vi "Replace Embedded SVG.vi"(7 "image":T1, 8 "error in":errorcluster, 9 "xlink:href":string, 10 "XML In":string, 11 "SVGImage in":refnum<class "SVGImage.lvclass">) -> (0 "error out":errorcluster, 2 "Edited XML Out":string, 3 "SVGImage out":refnum<class "SVGImage.lvclass">)   [LabVIEW 2019, in "SVGImage.lvclass"]
uses:
  SVGImage.lvclass
  ParseXML/Image.ctl
  SVGImage.lvclass/SVGImage.ctl
  EditSVG/EditSVG.lvclass
  ParseXML/ParseSVG.lvclass
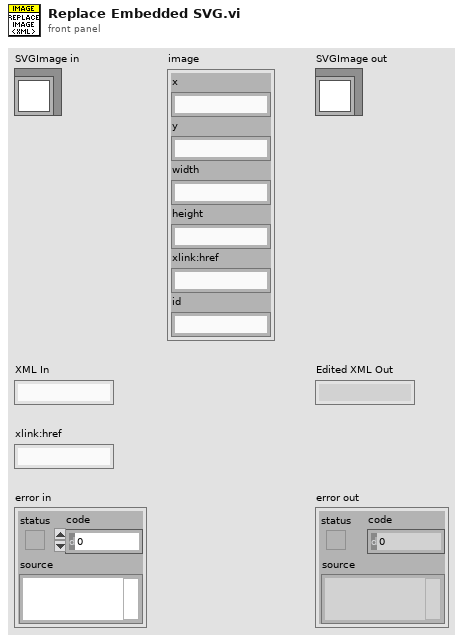
[diagram p1: front panel]
types:
  T1 = typedef "ParseSVG.lvclass/Image.ctl" = cluster{"x":string, "y":string, "width":string, "height":string, "xlink:href":string, "id":string}
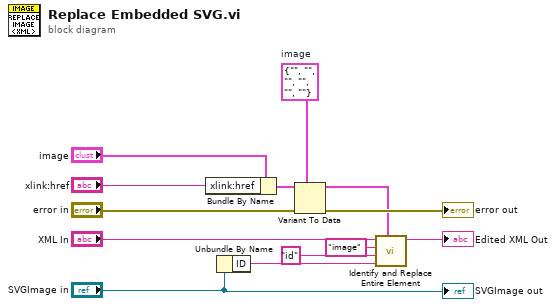
[diagram p0: block diagram]
diagram:
  w13 = T1 {"x"="", "y"="", "width"="", "height"="", "xlink:href"="", "id"=""}  # image
  n1 = Bundle By Name(cluster="image", "xlink:href"="xlink:href") -> (w6:T1)
  n2 = Unbundle By Name("SVGImage in") -> ("ID"=w4:string)
  n3 = Variant To Data(error in="error in", type=w13, Variant=w6) -> (data=w1:T1, error out=→"error out":errorcluster)
  n4 = call "Identify and Replace Entire Element.vi"("Named Cluster"=w1, "Identifying Attribute Value"=w4, "Identifying Attribute Type"="id", "Element Type"="image", "XML String"="XML In") -> ("Edited XML"=→"Edited XML Out":string)  [unwired: 6 in]
  "SVGImage out" <- "SVGImage in"
